vi "TargetSelect.vi"(11 "Target Info":T1(array[cluster])) -> (1 "Distance (ft)":dbl, 2 "Position.Y":dbl, 3 "Position.X":dbl)   [LabVIEW 2011]
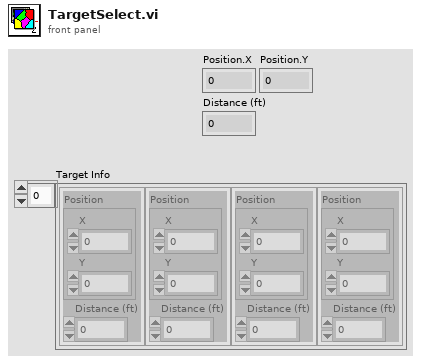
[diagram p1: front panel]
types:
  T1 = cluster{"Position":cluster{"X":dbl, "Y":dbl}, "Distance (ft)":dbl}[]
  T2 = cluster{"Target Info[0]":cluster{"Position":cluster{"X":dbl, "Y":dbl}, "Distance (ft)":dbl}, "Target Info[1]":cluster{"Position":cluster{"X":dbl, "Y":dbl}, "Distance (ft)":dbl}, "Target Info[2]":cluster{"Position":cluster{"X":dbl, "Y":dbl}, "Distance (ft)":dbl}, "Target Info[3]":cluster{"Position":cluster{"X":dbl, "Y":dbl}, "Distance (ft)":dbl}, "Target Info[4]":cluster{"Position":cluster{"X":dbl, "Y":dbl}, "Distance (ft)":dbl}, "Target Info[5]":cluster{"Position":cluster{"X":dbl, "Y":dbl}, "Distance (ft)":dbl}, "Target Info[6]":cluster{"Position":cluster{"X":dbl, "Y":dbl}, "Distance (ft)":dbl}, "Target Info[7]":cluster{"Position":cluster{"X":dbl, "Y":dbl}, "Distance (ft)":dbl}, "Target Info[8]":cluster{"Position":cluster{"X":dbl, "Y":dbl}, "Distance (ft)":dbl}}
  T3 = cluster{"Position":cluster{"X":dbl, "Y":dbl}, "Distance (ft)":dbl}
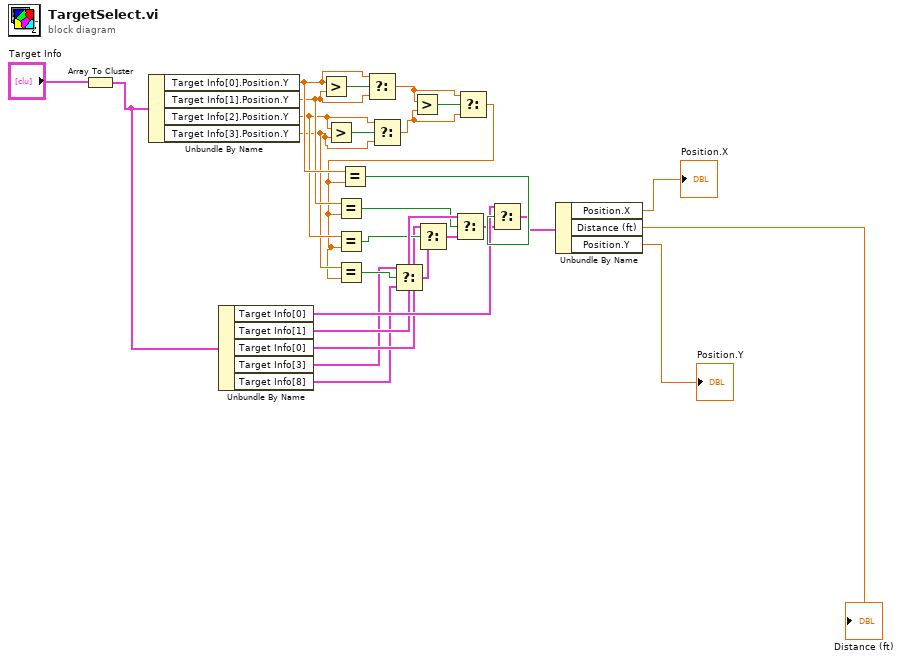
[diagram p0: block diagram]
diagram:
  n1 = Array To Cluster(array="Target Info") -> (cluster=w6:T2)
  n2 = Unbundle By Name(w6) -> ("Target Info[0].Position.Y"=w22:dbl, "Target Info[1].Position.Y"=w21:dbl, "Target Info[2].Position.Y"=w20:dbl, "Target Info[3].Position.Y"=w19:dbl)
  n3 = Unbundle By Name(w6) -> ("Target Info[0]"=w16:T3, "Target Info[1]"=w14:T3, "Target Info[0]"=w10:T3, "Target Info[3]"=w7:T3, "Target Info[8]"=w5:T3)
  n4 = Greater?(x=w22, y=w21) -> (0:w27:bool)
  n5 = Greater?(x=w20, y=w19) -> (0:w26:bool)
  n6 = Select(t=w22, s=w27, f=w21) -> (s? t:f=w24:dbl)
  n7 = Select(t=w20, s=w26, f=w19) -> (s? t:f=w23:dbl)
  n8 = Greater?(x=w24, y=w23) -> (0:w25:bool)
  n9 = Select(t=w24, s=w25, f=w23) -> (s? t:f=w18:dbl)
  n10 = Equal?(x=w21, y=w18) -> (x = y?=w13:bool)
  n11 = Equal?(x=w20, y=w18) -> (x = y?=w11:bool)
  n12 = Equal?(x=w19, y=w18) -> (x = y?=w8:bool)
  n13 = Equal?(x=w22, y=w18) -> (x = y?=w17:bool)
  n14 = Select(t=w7, s=w8, f=w5) -> (s? t:f=w9:T3)
  n15 = Select(t=w10, s=w11, f=w9) -> (s? t:f=w12:T3)
  n16 = Select(t=w14, s=w13, f=w12) -> (s? t:f=w15:T3)
  n17 = Select(t=w16, s=w17, f=w15) -> (s? t:f=w4:T3)
  n18 = Unbundle By Name(w4) -> ("Position.X"=→"Position.X":dbl, "Distance (ft)"=→"Distance (ft)":dbl, "Position.Y"=→"Position.Y":dbl)
